vi "Generate all noise.vi"(4 "lo cutoff":dbl, 6 "hi cutoff":dbl, 8 "start amplitude":dbl, 9 "end amplitude":dbl, 10 "sampling freq":dbl, 11 "samples":dbl) -> (3 "noise":dbl[](array[numeric]))   [LabVIEW 2012]
uses:
  <vilib>/Analysis/3filter.llb/Filter Passband Type.ctl
  <vilib>/Analysis/1siggen.llb/Ramp Pattern by Samples.vi
  <vilib>/Analysis/3filter.llb/Butterworth Filter (DBL).vi
  <vilib>/Analysis/NI_AALBase.lvlib
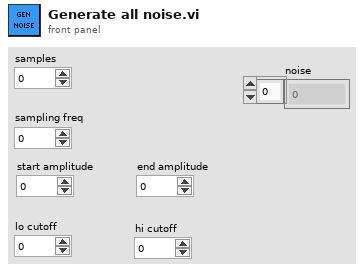
[diagram p1: front panel]
types:
  T1 = typedef "NI_AALBase.lvlib/Filter Passband Type.ctl" = enum32{"Lowpass", "Highpass", "Bandpass", "Bandstop"}
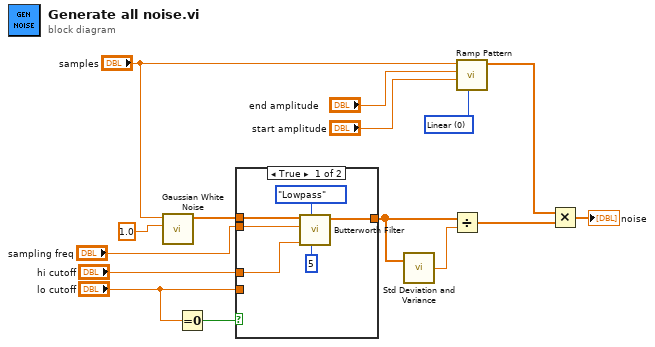
[diagram p0: block diagram]
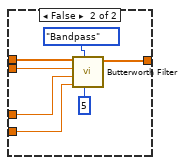
[diagram p2: hidden frame]
diagram:
  w4 = u16 0 items=["Linear", "Logarithmic"] ("type")
  n1 = call <vilib>:"Gaussian White Noise.vi"("standard deviation"=1.0, "samples"="samples") -> ("Gaussian noise pattern"=w13:dbl[])  [unwired: 8 in, 1 out]
  n2 = Equal To 0?(x="lo cutoff") -> (x = 0?=w11:bool)
  n3 = case shown="True" w11 {
    tunnel: "lo cutoff" -> [_ w23]
    tunnel: "hi cutoff" -> [w18 w24]
    tunnel: "sampling freq" -> [w20 w27]
    tunnel: w13 -> [w19 w26]
    tunnel: [w16 w22] -> w9
    frame True {
      n4 = call-poly <vilib>:"Butterworth Filter.vi"("order"=5, "filter type"=Filter_Passband_Type."Lowpass", "low cutoff freq: fl"=w18, "sampling freq: fs"=w20, "X"=w19) -> ("Filtered X"=w16:dbl[])  [unwired: 3 in, 1 out]
    }
    frame False {
      n5 = call-poly <vilib>:"Butterworth Filter.vi"("order"=5, "filter type"=Filter_Passband_Type."Bandpass", "low cutoff freq: fl"=w23, "high cutoff freq: fh"=w24, "sampling freq: fs"=w27, "X"=w26) -> ("Filtered X"=w22:dbl[])  [unwired: 2 in, 1 out]
    }
  }
  n6 = call <vilib>:"Std Deviation and Variance.vi"("X"=w9) -> ("standard deviation"=w8:dbl)  [unwired: 1 in, 2 out]
  n7 = Divide(x=w9, y=w8) -> (x/y=w3:dbl[])
  n8 = call-poly <vilib>:"Ramp Pattern.vi"("type"=w4, "start"="start amplitude", "end"="end amplitude", "samples"="samples") -> ("Ramp Pattern"=w2:dbl[])  [unwired: 6 in, 1 out]
  n9 = Multiply(x=w2, y=w3) -> (x*y=→"noise":dbl[])
